vi "Set_Speed.vi"(5 "Channel Name (Calib Tweak)":string, 6 "Calib Tweak":dbl format="%.2f", 7 "Client Name":string, 8 "Channel Name (Volts/Amps)":string, 9 "Demanded Velocity":dbl format="%.2f", 10 "Channel Name (Velocity)":string) -> (0 "Errors":string)   [LabVIEW 2021]
uses:
  ADAM Client/Sub VIs/ADAM Controls/Update_scan_value.ctl
panel:
  out "TweakedDemand":dbl
  out "Demand":dbl
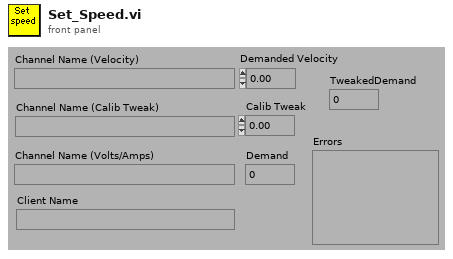
[diagram p1: front panel]
types:
  T1 = typedef "Update_scan_value.ctl" = cluster{"Channel Name":string, "New Value":dbl, "!Auto_Off":bool}
  T2 = enum16{"Append to Global", "Read Global then Clear"}
  T3 = typedef "Ch_description_ADAM.ctl" = cluster{"Ch Name":string, "Type":T4, "Function":T5, "Ch State":T6, "Calibration type":T7, "A":dbl, "B":dbl, "C":dbl, "D":dbl, "Comments":string, "Address":T8, "String":string, "Duty":u16}
  T4 = typedef "Module_type_ADAM.ctl" = string
  T5 = typedef "Function_ADAM.ctl" = enum16{"Analogue Input", "Digital Input", "Event counter", "Event rate", "Analogue Output", "Digital Output", "Relay Output"}
  T6 = typedef "Channel_State.ctl" = enum16{"On", "Off", "Always On", "Always Off"}
  T7 = typedef "Calib_type_ADAM.ctl" = string
  T8 = typedef "Address.ctl" = cluster{"Main":i32, "Ch.":i32, "Sub":i32, "Port Name":string}
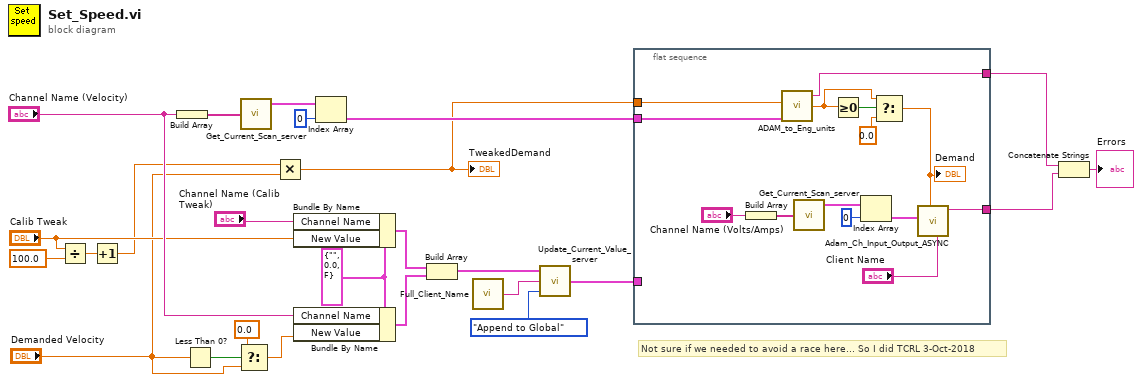
[diagram p0: block diagram]
diagram:
  w8 = T1 {"Channel Name"="", "New Value"=0.0, "!Auto_Off"=FALSE} ("Update Scan Value Cluster")
  # "Not sure if we needed to avoid a race here... So I did TCRL 3-Oct-2018"
  n1 = Divide(x="Calib Tweak", y=100.0) -> (x/y=w15:dbl)
  n2 = Increment(x=w15) -> (x+1=w13:dbl)
  n3 = Build Array("Channel Name (Velocity)") -> (w23:string[])
  n4 = Less Than 0?(x="Demanded Velocity") -> (x < 0?=w20:bool)
  n5 = Select(t=0.0, s=w20, f="Demanded Velocity") -> (s? t:f=w14:dbl)
  n6 = call "Get_Current_Scan_server.vi"("Desired Channels"=w23) -> ("Ch Description Array"=w25:T3[])  [unwired: 2 out]
  n7 = Multiply(x=w13, y="Demanded Velocity") -> (x*y=w5:dbl)
  "TweakedDemand" <- w5
  n8 = Bundle By Name(cluster=w8, "Channel Name"="Channel Name (Calib Tweak)", "New Value"="Calib Tweak") -> (w17:T1)
  n9 = Bundle By Name(cluster=w8, "Channel Name"="Channel Name (Velocity)", "New Value"=w14) -> (w22:T1)
  n10 = Index Array(array=w25, index=0) -> (element=w6:T3)
  n11 = Build Array(w17, w22) -> (w21:T1[])
  n12 = call "Full_Client_Name.vi"() -> ("Client Name"=w19:string)
  n13 = call "Update_Current_Value_server.vi"("Mode"=T2."Append to Global", "Client HD name"=w19, "Update array in"=w21) -> ("Update array out"=w4:T1[])
  n14 = flat-sequence {
    tunnel: w6 -> [w29]
    tunnel: w5 -> [w28]
    tunnel: w4 -> [_]
    tunnel: [w27] -> w3
    tunnel: [w26] -> w2
    frame #0 {
      n15 = Build Array("Channel Name (Volts/Amps)") -> (w32:string[])
      n16 = call "ADAM_to_Eng_units.vi"("Ch Description"=w29, "Raw"=w28) -> ("Calibrated units"=w36:dbl, "Comments"=w27:string)  [unwired: 3 out]
      n17 = call "Get_Current_Scan_server.vi"("Desired Channels"=w32) -> ("Ch Description Array"=w33:T3[])  [unwired: 2 out]
      n18 = Greater Or Equal To 0?(x=w36) -> (x >= 0?=w35:bool)
      n19 = Index Array(array=w33, index=0 ("Index")) -> (element=w34:T3)
      n20 = Select(t=w36, s=w35, f=0.0) -> (s? t:f=w37:dbl)
      "Demand" <- w37
      n21 = call "Adam_Ch_Input_Output_ASYNC.vi"("Client Name"="Client Name", "Value to Output"=w37, "Ch Description"=w34) -> ("Scan comment"=w26:string)  [unwired: 4 in, 4 out]
    }
  }
  n22 = Concatenate Strings(w3, w2) -> (→"Errors":string)
